vi "New Parameters Event.vi"() -> (3 "New Parameters":refnum<user-event>)   [LabVIEW 2020]
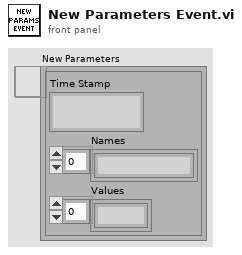
[diagram p1: front panel]
types:
  T1 = cluster{"Time Stamp":timestamp, "Names":string[], "Values":dbl[]}
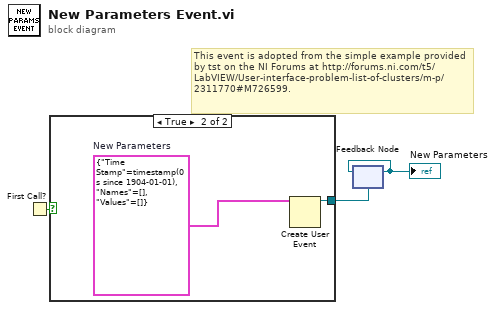
[diagram p0: block diagram]
diagram:
  # "This event is adopted from the simple example provided by tst on the NI Forums at http://forums.ni.com/t5/LabVIEW/User-interface-problem-list-of-clusters/m-p/2311770#M726599."
  n1 = First Call?() -> (First Call?: T/F=w3:bool)
  n2 = case shown="True" w3 {
    tunnel: [_ w5] -> w2
    frame False {
    }
    frame True {
      w4 = T1 {"Time Stamp"=timestamp(0 s since 1904-01-01), "Names"=[], "Values"=[]}  # New Parameters
      n3 = Create User Event(user event datatype=w4) -> (user event=w5:refnum<user-event>)  [unwired: 1 in, 1 out]
    }
  }
  n4 = feedback #1(w2) -> (w1:refnum<user-event>)
  "New Parameters" <- w1
  n5 = feedback-in #1(w1) -> ()
